vi "Resolve Real Link.vi"(6 "Max Path Length":i32=255 min=0, 8 "Error In":errorcluster, 10 "Remote Link Path":string, 11 "SFTP In":refnum<class "SFTP.lvclass">) -> (0 "Error Out":errorcluster, 2 "Remote Source Path":string, 3 "SFTP Out":refnum<class "SFTP.lvclass">)   [LabVIEW 2021, in "Field_RnD_Services_LIBSSH2_Toolkit.lvlib" / "SFTP.lvclass"]
doc: "Gets the absolute path of a real link's target, or source, on the remote SFTP server."
uses:
  SFTP.lvclass
  SFTP.lvclass/SFTP.ctl
  Field_RnD_Services_LIBSSH2_Toolkit.lvlib
  Session/Session.lvclass
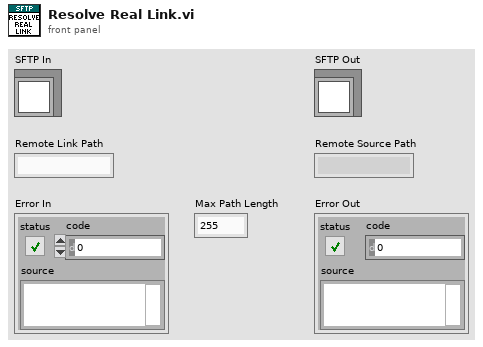
[diagram p1: front panel]
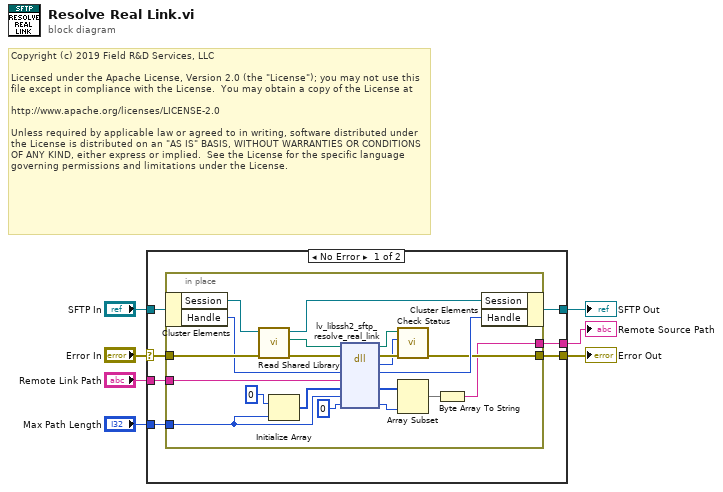
[diagram p0: block diagram]
diagram:
  # "Copyright (c) 2019 Field R&D Services, LLC\n\nLicensed under the Apache License, Version 2.0 (the \"License\"); you may not use this file except in compliance with the License.  You may obtain a copy of the License at\n\nhttp://www.apache.org/licenses/LICENSE-2.0\n\nUnless required by applicable law or agreed to in writing, software distributed under the License is distributed on an \"AS IS\" BASIS, WITHOUT WARRANTIES OR CONDITIONS OF ANY KIND, either express or implied.  See the License for the specific language governing permissions and limitations under the License."
  n1 = case shown="No Error" "Error In" {
    selector: "Error In" -> [w14 w36]
    tunnel: [w13 w36] -> w6
    tunnel: "SFTP In" -> [w12 w35]
    tunnel: [w11 w35] -> w4
    tunnel: "Remote Link Path" -> [w10 _]
    tunnel: "Max Path Length" -> [w9 _]
    tunnel: [w8 _] -> w1
    frame No Error {
      n2 = in-place {
        in-place-border: w14 -> [w29]
        in-place-border: [w30] -> w13
        in-place-border: w10 -> [w23]
        in-place-border: w9 -> [w20]
        in-place-border: [w15] -> w8
        n3 = in-place-cluster #1(w12) -> ("Session"=w28:refnum<class "Session.lvclass">, "Handle"=w24:u64)
        n4 = call "Read Shared Library.vi"("Error In"=w29, "Session In"=w28) -> ("Erorr Out"=w26:errorcluster, "libssh2lv Shared Library"=w25:path, "Session Out"=w27:refnum<class "Session.lvclass">)  [unwired: 7 in]
        n5 = Initialize Array(u8 0, w20) -> (w21:u8[])
        n6 = dll-call lib="libssh2lv.*" fn="lv_libssh2_sftp_resolve_real_link"(path in=w25, error in=w26, "handle"=w24, "link_path"=w23, "source_path"=w21, "source_path_max_length"=w20, "read_count"=u64 0) -> (path out=w32:path, error out=w33:errorcluster, "status"=w31:i32, "handle"=w34:u64, "source_path"=w18:u8[], "read_count"=w17:u64)  [unwired: 3 in]
        n7 = call "Check Status.vi"("Error In"=w33, "Status"=w31, "libssh2lv Shared Library In"=w32) -> ("Error Out"=w30:errorcluster)  [unwired: 7 in, 1 out]
        n8 = Array Subset(array=w18, length=w17) -> (w16:u8[])  [unwired: 1 in]
        n9 = Byte Array To String(unsigned byte array=w16) -> (string=w15:string)
        n10 = in-place-cluster #1("Session"=w27, "Handle"=w34) -> (w11:refnum<class "SFTP.lvclass">)
      }
    }
    frame Error {
    }
  }
  "Error Out" <- w6
  "SFTP Out" <- w4
  "Remote Source Path" <- w1
